vi "Bit_to_Boolean.vi"(1 "Bit In":u32 max=1) -> (0 "Boolean Out":bool)   [LabVIEW 2011]
doc: "This vi converts a logic 0 or 1 input to a true or false Boolean."
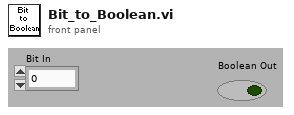
[diagram p1: front panel]
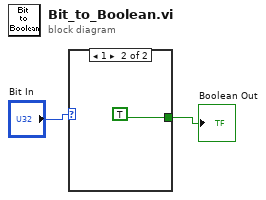
[diagram p0: block diagram]
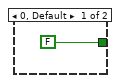
[diagram p2: hidden frame]
diagram:
  n1 = case shown="1" "Bit In" {
    tunnel: [FALSE TRUE] -> w1
    frame 0, Default {
    }
    frame 1 {
    }
  }
  "Boolean Out" <- w1
